vi "TEST Report Class.vi"() -> ()   [LabVIEW 2009, in "Report.lvclass"]
doc: "This VI simply tests basic operation of the overall class hierarchy.\n\nAAL 9/09"
uses:
  Report.lvclass
  Plug Ins/XML Report Class/XML Report.lvclass
panel:
  in  "Header":string
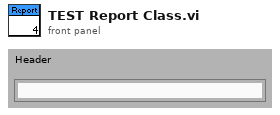
[diagram p1: front panel]
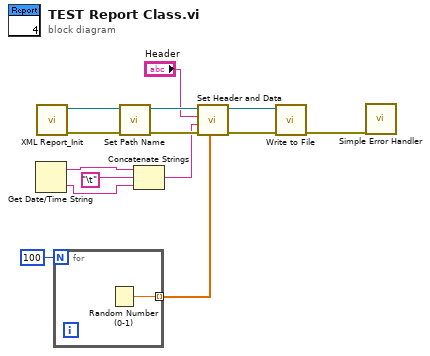
[diagram p0: block diagram]
diagram:
  n1 = Get Date/Time String() -> (date string=w8:string, time string=w6:string)  [unwired: 3 out]
  n2 = call "XML Report_Init.vi"() -> ("error out"=w1:errorcluster, "XML_Report out"=w2:refnum<class "XML Report.lvclass">)  [unwired: 1 in, 9 out]
  n3 = for {
    N: 100 -> [_]
    tunnel: [w15] -> w4 mode=indexing
    n4 = Random Number (0-1)() -> (number: 0 to 1=w15:dbl)
  }
  n5 = call-dynamic "Set Path Name.vi"("error in (no error)"=w1, "Report"=w2) -> ("error out"=w12:errorcluster, "Report out"=w14:refnum<class "XML Report.lvclass">)  [unwired: 1 in, 7 out]
  n6 = Concatenate Strings(w8, "\t", w6) -> (w5:string)
  n7 = call-dynamic "Set Header and Data.vi"("Data Array"=w4, "error in (no error)"=w12, "Data & Time String"=w5, "Header"="Header", "Report"=w14) -> ("error out"=w11:errorcluster, "Report out"=w13:refnum<class "XML Report.lvclass">)  [unwired: 5 out]
  n8 = call-dynamic "Write to File.vi"("error in (no error)"=w11, "XML Report"=w13) -> ("error out"=w10:errorcluster)  [unwired: 9 out]
  n9 = call <vilib>:"Simple Error Handler.vi"("error in (no error)"=w10) -> ()  [unwired: 1 in, 8 out]
